vi "Common Device Queue Get Command.vi"(0 "Common Queue":refnum<queue>, 11 "Notifier Name":string) -> (4 "Common Queue":refnum<queue>, 8 "Command":string)   [LabVIEW 2025]
panel:
  out "Queue Element":string
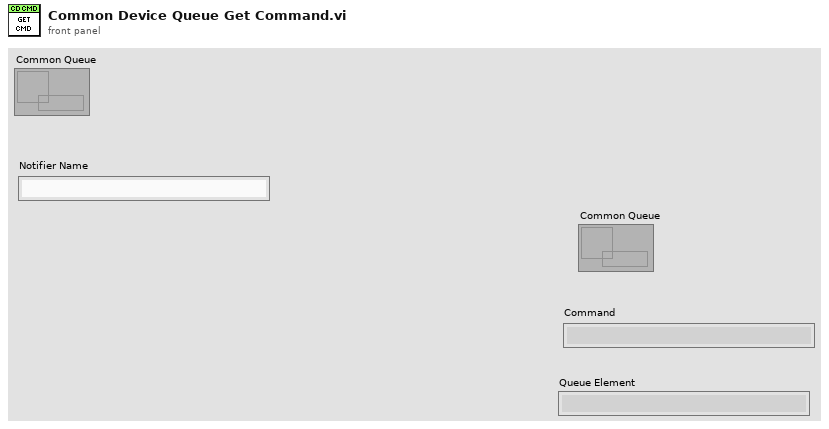
[diagram p1: front panel]
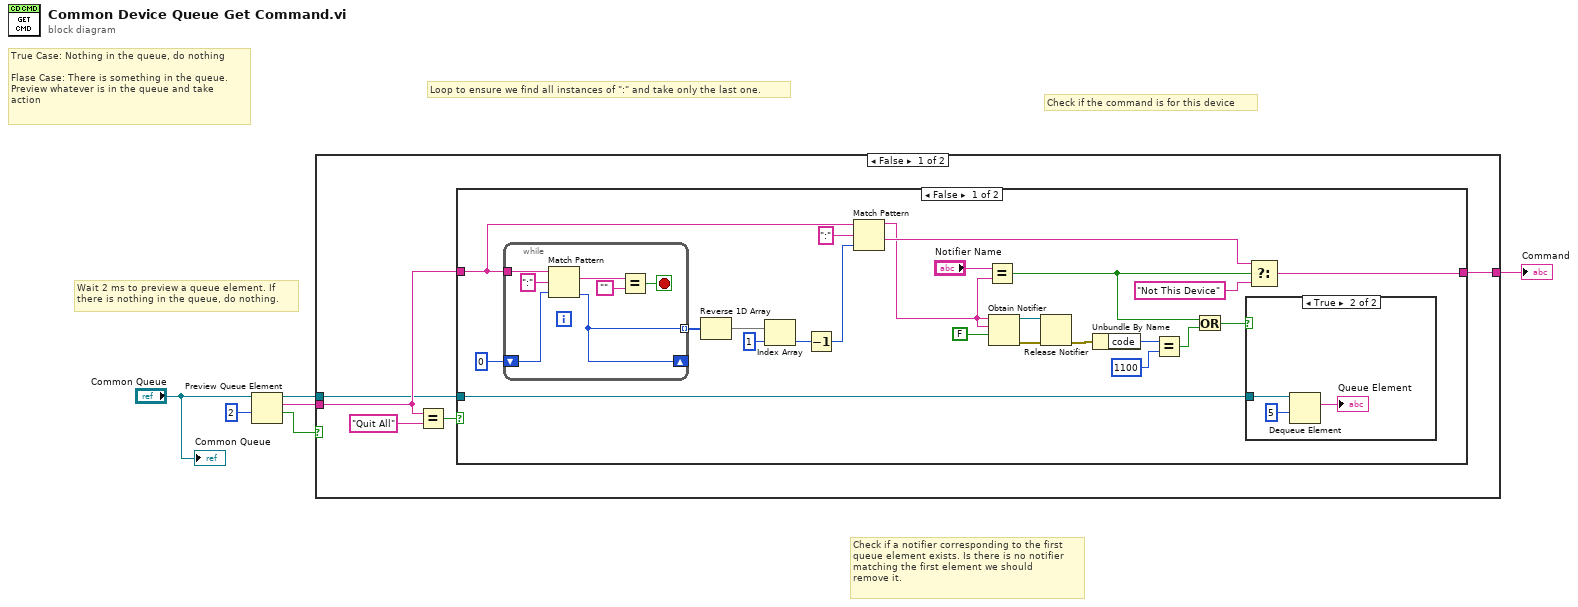
[diagram p0: block diagram]
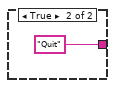
[diagram p3: hidden frame]
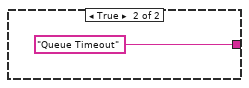
[diagram p4: hidden frame]
diagram:
  # "Loop to ensure we find all instances of \":\" and take only the last one."
  # "True Case: Nothing in the queue, do nothing\n\nFlase Case: There is something in the queue.\nPreview whatever is in the queue and take\naction"
  # "Wait 2 ms to preview a queue element. If\nthere is nothing in the queue, do nothing."
  # "Check if a notifier corresponding to the first\nqueue element exists. Is there is no notifier\nmatching the first element we should\nremove it."
  # "Check if the command is for this device"
  n1 = Preview Queue Element(queue="Common Queue", timeout in ms (-1)=2) -> (queue out=w4:refnum<queue>, element=w5:string, timed out?=w1:bool)  [unwired: 1 in, 1 out]
  n2 = case shown="False" w1 {
    tunnel: [w11 "Queue Timeout" ("t")] -> w6
    tunnel: w5 -> [w8 _]
    tunnel: w4 -> [w7 _]
    frame False {
      n3 = Equal?(x=w8, y="Quit All" ("regular expression")) -> (x = y?=w9:bool)
      n4 = case shown="False" w9 {
        tunnel: w7 -> [w27 _]
        tunnel: [w26 "Quit" ("t")] -> w11
        tunnel: w8 -> [w14 _]
        frame False {
          n5 = while {
            shift-right: [w35] -> _
            shift-left: 0 -> [w37]
            tunnel: w14 -> [w36]
            tunnel: [w35] -> w18 mode=indexing
            stop <- w38 stop-if-true
            n6 = Match Pattern(string=w36, regular expression=":", offset (0)=w37) -> (match substring=w40:string, offset past match=w35:i32)  [unwired: 2 out]
            n7 = Equal?(x=w40, y="") -> (x = y?=w38:bool)
          }
          n8 = Reverse 1D Array(array=w18) -> (reversed array=w19:i32[])
          n9 = Index Array(array=w19, index=1) -> (element=w20:i32)
          n10 = Decrement(x=w20) -> (x-1=w21:i32)
          n11 = Match Pattern(string=w14, regular expression=":" ("search string/char (-)"), offset (0)=w21) -> (before substring=w12:string, after substring=w13:string)  [unwired: 2 out]
          n12 = Equal?(x="Notifier Name", y=w12) -> (x = y?=w32:bool)
          n13 = Obtain Notifier(name (unnamed)=w12, notification data type=w12, create if not found? (T)=FALSE) -> (notifier out=w25:refnum<notifier>, error out=w24:errorcluster)  [unwired: 1 in, 1 out]
          n14 = Release Notifier(notifier=w25, error in (no error)=w24) -> (error out=w23:errorcluster)  [unwired: 1 in, 2 out]
          n15 = Unbundle By Name(w23) -> ("code"=w31:i32)
          n16 = Equal?(x=w31, y=1100) -> (x = y?=w33:bool)
          n17 = Or(x=w32, y=w33) -> (x .or. y?=w34:bool)
          n18 = case shown="True" w34 {
            tunnel: w27 -> [_ w42]
            frame False {
            }
            frame True {
              n19 = Dequeue Element(queue=w42, timeout in ms (-1)=5) -> (element=→"Queue Element":string)  [unwired: 1 in, 3 out]
            }
          }
          n20 = Select(t=w13, s=w32, f="Not This Device") -> (s? t:f=w26:string)
        }
        frame True {
        }
      }
    }
    frame True {
    }
  }
  "Command" <- w6
  "Common Queue" <- "Common Queue"
